vi "ProcessCommand.vi"(5 "Ctl Refnum":refnum<vi>, 7 "Command":variant, 8 "error in (no error)":errorcluster, 9 "Data":T1=variant(string "Default"), 10 "Queue with Cluster Reference":T2, 11 "Shell Command in":refnum<class "Shell Command.lvclass">) -> (0 "error out":errorcluster, 2 "Queue (dup)":T2, 3 "Shell Command out":refnum<class "Shell Command.lvclass">)   [LabVIEW 2010, in "Shell Command.lvclass"]
doc: "This VI serves as the dynamic dispatch VI for Shell Command objects. The items are cued up with the prefix of \"Command - \".\n\nInputs:\nShell Command in - object used for commands from the shell\nCommand - SignalCommandControl typedef\nQueue with Cluster Reference - reference to the EVM queue for inserting commands\nCtl Refnum - no valid for this VI\nData - variant type; any data needed to pass to processing loop\nerror in - error input cluster\n\nOutputs:\nEVM Command out - input object passed through\nQueue (dup) - input queue reference passed through\nerror out - error output cluster"
uses:
  Shell Command.lvclass
  <userlib>/Common/Queue with Cluster/TYP_Queue with Cluster Reference.ctl
  Controls/TYP_VariantDefault.ctl
  adcpro_v2/pdk_lib/libadcpro/SignalPlugin/controls/SignalPluginCommand.ctl
  Shell Command.lvclass/Shell Command.ctl
  <userlib>/Common/Queue with Cluster/Enqueue - ClusterBoth.vi
  adcpro_v2/pdk_lib/libadcpro/SignalPlugin/SignalPlugin.lvclass
panel:
  # "Inputs"
  # "Outputs"
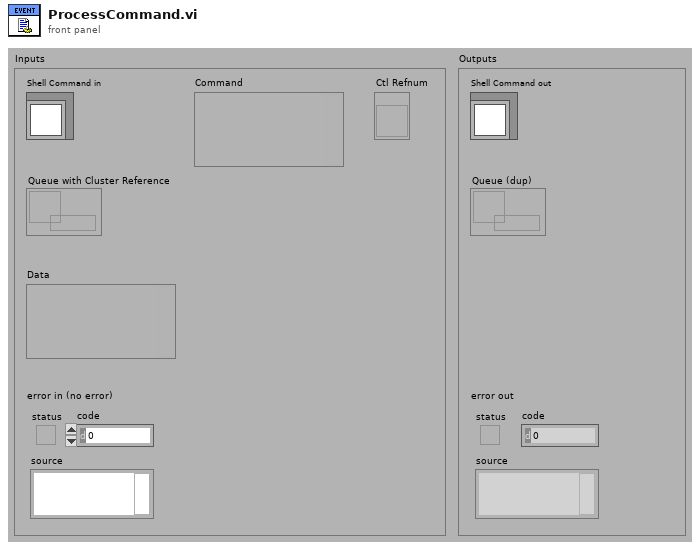
[diagram p1: front panel]
types:
  T1 = typedef "TYP_VariantDefault.ctl" = variant
  T2 = typedef "TYP_Queue with Cluster Reference.ctl" = refnum<queue>
  T3 = typedef "libadcpro.lvlib/SignalPlugin.lvclass/SignalPluginCommand.ctl" = enum16{"None", "Load", "Unload", "<not used>", "Acquire", "Stop", "SamplesAvailable"}
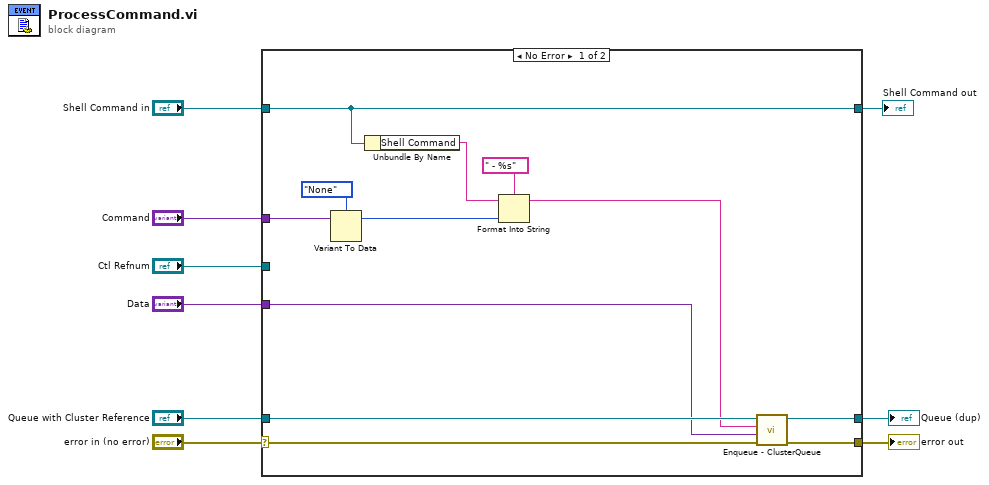
[diagram p0: block diagram]
diagram:
  n1 = case shown="No Error" "error in (no error)" {
    selector: "error in (no error)" -> [w19 w24]
    tunnel: [w18 w24] -> w8
    tunnel: [w15 w23] -> w6
    tunnel: "Shell Command in" -> [w15 w23]
    tunnel: "Command" -> [w21 _]
    tunnel: [w17 w22] -> w3
    tunnel: "Queue with Cluster Reference" -> [w16 w22]
    tunnel: "Ctl Refnum" -> [_ _]
    tunnel: "Data" -> [w10 _]
    frame No Error {
      n2 = Variant To Data(Variant=w21, type=SignalPluginCommand."None" ("NewVal")) -> (data=w14:T3)  [unwired: 1 in, 1 out]
      n3 = Unbundle By Name(w15) -> ("Shell Command"=w13:string)
      n4 = Format Into String(format string=" - %s", initial string=w13, w14) -> (resulting string=w11:string)  [unwired: 1 in, 1 out]
      n5 = call-poly <userlib>:"Enqueue - ClusterQueue.vi"("error in (no error)"=w19, "Data"=w10, "Command"=w11, "Queue with Cluster Reference"=w16) -> ("error out"=w18:errorcluster, "Queue Out (dup)"=w17:T2)  [unwired: 6 in]
    }
    frame Error {
    }
  }
  "error out" <- w8
  "Shell Command out" <- w6
  "Queue (dup)" <- w3
